vi "PH_Beckhoff_PP_PU.ProcCases.vi"(0 "i ref in":refnum<vi>, 1 "selector":string, 2 "Data":T1, 3 "call cluster":T2={"Object"="", "Selector"="", "CallType"=enum."synchronous", "Async Object"="", "Async Selector"="", "Data Descriptor"="", "Data"=[], "Error #"=0, "Expire"=0}, 5 "error in (no error)":errorcluster) -> (14 "i ref out":refnum<vi>, 17 "answer cluster":T2={"Object"="", "Selector"="", "CallType"=enum."synchronous", "Async Object"="", "Async Selector"="", "Data Descriptor"="", "Data"=[], "Error #"=0, "Expire"=0}, 19 "error out":errorcluster)   [LabVIEW 2014, in "PH_Beckhoff_PP_PU.lvlib"]
doc: "This method is called by a process from within the default case in the event loop. The methods of a class that are linked to events will be called from THIS method. Add your code here."
uses:
  PH_Beckhoff_PP_PU.lvlib
  CS_Core/CSSystem/CoreDefs/CoreDefs.call_type.ctl
  CS_Core/BaseProcess/BaseProcess.descriptor string definition.ctl
  CS_Core/CSSystem/CoreDefs/CoreDefs.rawDataType.ctl
  CS_Core/CSSystem/CoreLib/CoreLib.string 2 byte array.vi
  PH_Beckhoff/PH_Beckhoff.lvlib
  CS_Core/BaseProcess/BaseProcess.lvlib
  CS_Core/CSSystem/CoreLib/CoreLib.lvlib
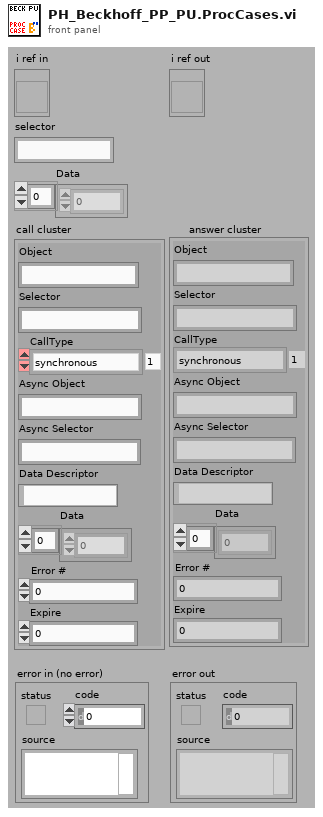
[diagram p1: front panel]
types:
  T1 = typedef "CoreDefs.rawDataType.ctl" = i8[]
  T2 = typedef "CoreDefs.call_type.ctl" = cluster{"Object":string, "Selector":string, "CallType":enum16{"simple", "synchronous", "asynchronous"}, "Async Object":string, "Async Selector":string, "Data Descriptor":T3, "Data":T1, "Error #":i32, "Expire":u32}
  T3 = typedef "BaseProcess.lvlib/BaseProcess.descriptor string definition.ctl" = string
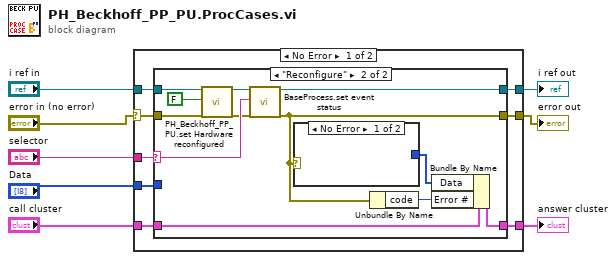
[diagram p0: block diagram]
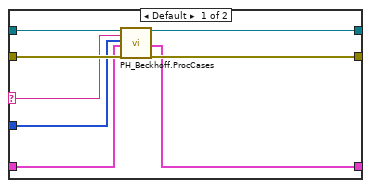
[diagram p2: hidden frame]
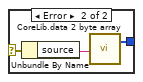
[diagram p3: hidden frame]
diagram:
  n1 = case shown="No Error" "error in (no error)" {
    selector: "error in (no error)" -> [w9 w40]
    tunnel: "selector" -> [w16 _]
    tunnel: [w15 w41] -> w7
    tunnel: "Data" -> [w14 _]
    tunnel: "call cluster" -> [w13 w41]
    tunnel: "i ref in" -> [w12 w42]
    tunnel: [w11 w42] -> w3
    tunnel: [w10 w40] -> w2
    frame No Error {
      n2 = case shown="\"Reconfigure\"" w16 {
        selector: w16 -> [w18 w31]
        tunnel: w14 -> [w19 _]
        tunnel: w12 -> [w17 w35]
        tunnel: [w24 w26] -> w11
        tunnel: w13 -> [w20 w30]
        tunnel: [w21 w29] -> w15
        tunnel: w9 -> [w23 w36]
        tunnel: [w22 w25] -> w10
        frame Default {
          n3 = call "PH_Beckhoff.ProcCases.vi"("i ref in"=w17, "selector"=w18, "Data"=w19, "call cluster"=w20, "error in (no error)"=w23) -> ("i ref out"=w24:refnum<vi>, "answer cluster"=w21:T2, "error out"=w22:errorcluster)  [unwired: 12 in]
        }
        frame "Reconfigure" {
          n4 = call "PH_Beckhoff_PP_PU.set Hardware reconfigured.vi"("i ref in"=w35, "Hardware reconfigured?"=FALSE, "error in"=w36) -> ("i ref out"=w28:refnum<vi>, "error out"=w27:errorcluster)  [unwired: 15 in]
          n5 = call "BaseProcess.set event status.vi"("i ref in"=w28, "EventStatus"=w31, "error in (no error)"=w27) -> ("i ref out"=w26:refnum<vi>, "error out"=w25:errorcluster)  [unwired: 14 in, 1 out]
          n6 = case shown="No Error" w25 {
            selector: w25 -> [_ w39]
            tunnel: [_ w37] -> w33
            frame No Error {
            }
            frame Error {
              n7 = Unbundle By Name(w39) -> ("source"=w38:string)
              n8 = call-poly "CoreLib.data 2 byte array.vi"("string"=w38) -> ("byteArray out"=w37:T1)  [unwired: 18 in]
            }
          }
          n9 = Unbundle By Name(w25) -> ("code"=w32:i32)
          n10 = Bundle By Name(cluster=w30, "Data"=w33, "Error #"=w32) -> (w29:T2)
        }
      }
    }
    frame Error {
    }
  }
  "answer cluster" <- w7
  "i ref out" <- w3
  "error out" <- w2
